vi "WVDIAL_1_AMCS_2.0_15m_res.vi"() -> ()   [LabVIEW 2012]
uses:
  <vilib>/Analysis/baseanly.llb/Mean (DBL).vi
  NCAR_DIAL_Labview/AMCS_Data.vi
  AmcsUsb.dll
  <vilib>/Analysis/NI_AALBase.lvlib
panel:
  out "x/y":dbl=nan
  out "Narrow Ratio":dbl(graph)=nan
  in  "Near Ch Offline mult":dbl=0.85
  out "size(s)":i32=5601
  in  "Channels":u32=4
  in  "Data Reads":i32=4
  out "Loop Count":i32=11
  in  "TC Start":i32=2 min=1 max=1894
  in  "TC Length":i32=15 min=2 max=280
  out "TC background sub over length":cluster{dbl, dbl, dbl, dbl}(graph)={0.0, 0.0, 1715.36170212766, 71287.61702127659}
  out "return type":i32
  out "Raw Uncorrected Return":u16[][](graph)
  in  "stop":bool
  out "Corrected Return":dbl[][](graph) caption="Corrected Signal"
  out "Max. Rep. Rate (Hz)":dbl=7091.695624423801
  out "Data Collection Time per Column":dbl=2.00004285
  out "Minimum Sync Pulse Period(µs)":dbl=141.01 format="%.2f"
  in  "y units":u16(ring) items=["Bin #", "Sampling Time(µs)", "Range(m)"]
  in  "Time Resolution Per Bin(ns)":u16=100 min=5 max=1063 step=1
  in  "Number of Accumulates":u32=14285 min=1 max=32767 step=1
  in  "Pulse A Polarity":enum16{"Low", "High"}(ring)=enum."High"
  in  "Sync Pulse Polarity":enum32{"Low", "High"}(ring)=enum."High"
  in  "Accumulation Delay(ns)":u16=10 min=10 max=1270 step=1
  in  "Pulse B Delay(ns)":u32=170000 min=80 max=327600 step=1
  in  "Pulse A Delay(ns)":u32=1040 min=80 max=327600
  in  "bins":u32=1400 min=2 max=4095 step=1
  out "y offset":u16=10
  in  "ns scale":u16=100
  in  "Pulse B Polarity":enum16{"Low", "High"}(ring)=enum."High"
  out "Running?":bool
  out "Device ID":u32
  out "Open?":bool=TRUE
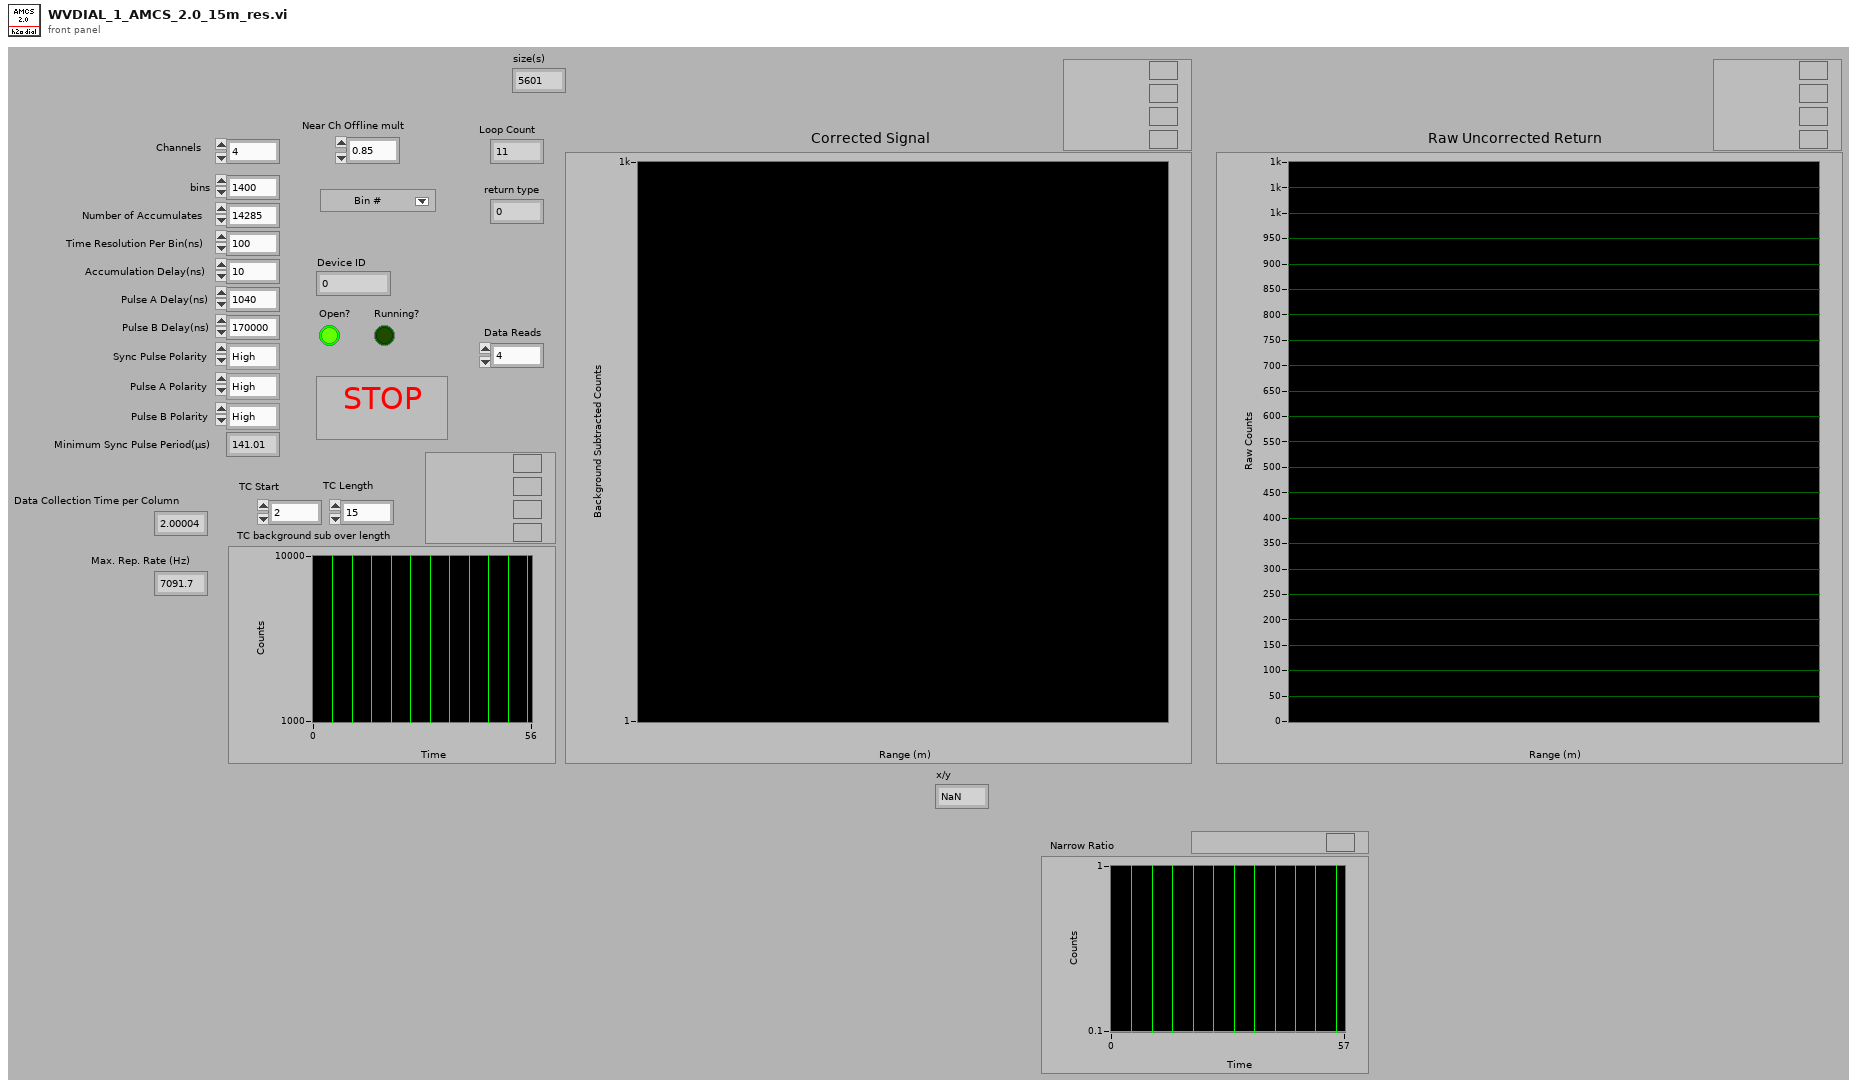
[diagram p1: front panel]
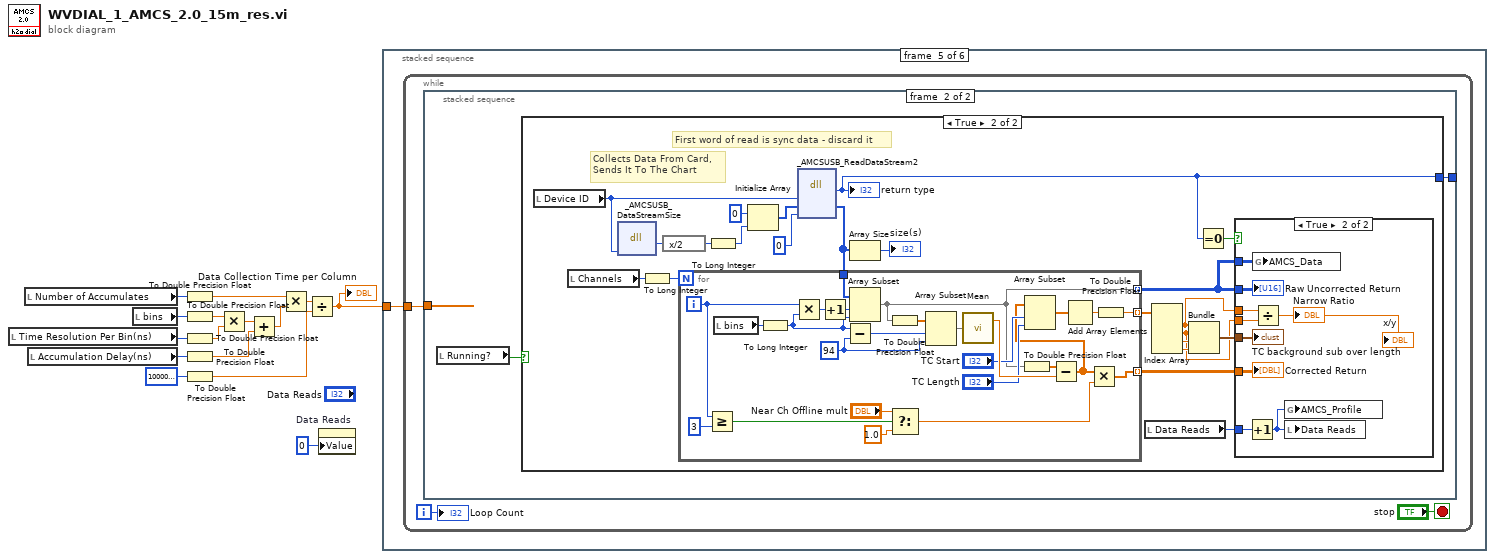
[diagram p0: block diagram]
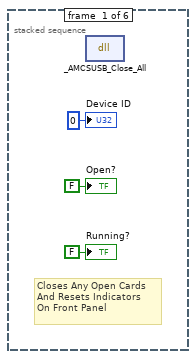
[diagram p2: hidden frame]
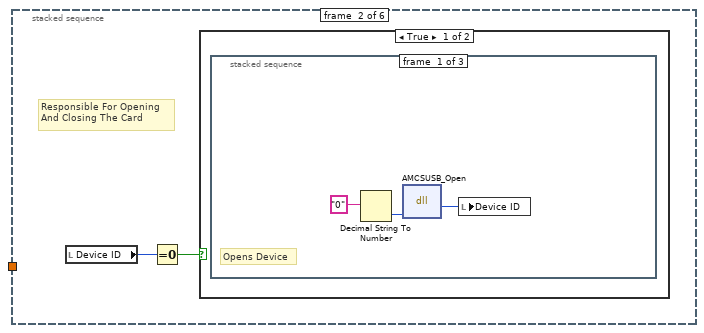
[diagram p3: hidden frame]
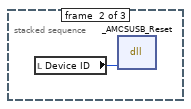
[diagram p4: hidden frame]
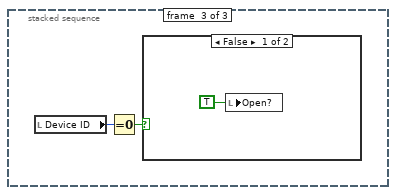
[diagram p5: hidden frame]
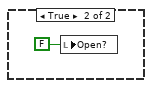
[diagram p6: hidden frame]
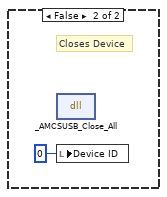
[diagram p7: hidden frame]
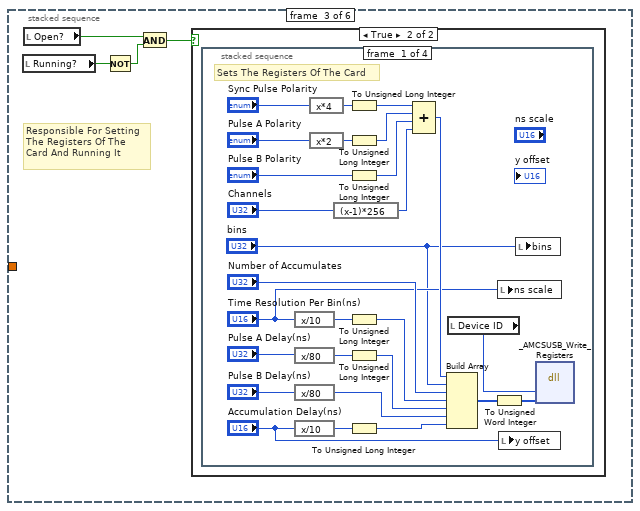
[diagram p8: hidden frame]
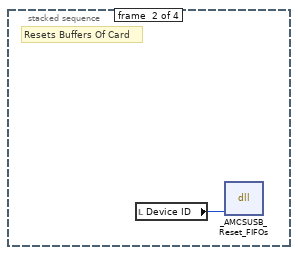
[diagram p10: hidden frame]
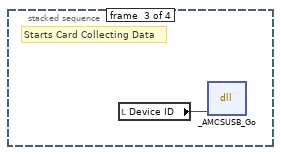
[diagram p11: hidden frame]
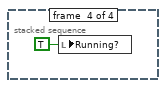
[diagram p12: hidden frame]
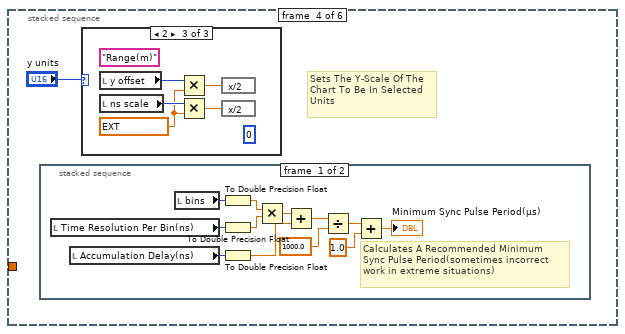
[diagram p13: hidden frame]
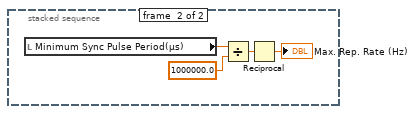
[diagram p14: hidden frame]
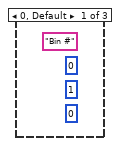
[diagram p15: hidden frame]
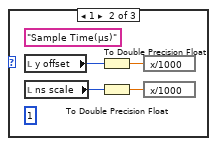
[diagram p16: hidden frame]
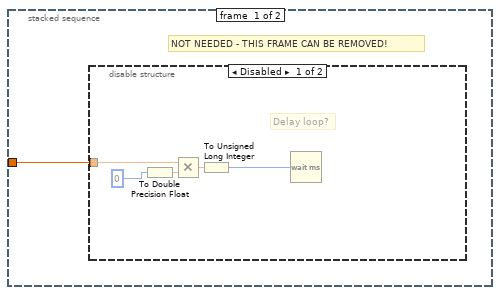
[diagram p17: hidden frame]
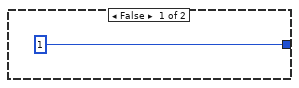
[diagram p19: hidden frame]
diagram:
  n1 = local read "Time Resolution Per Bin(ns)"() -> (w4:u16)
  n2 = local read "Number of Accumulates"() -> (w11:u32)
  n3 = local read "Accumulation Delay(ns)"() -> (w2:u16)
  n4 = local read "bins"() -> (w6:u32)
  n5 = To Double Precision Float(number=w11) -> (double precision float=w10:dbl)
  n6 = To Double Precision Float(number=w6) -> (double precision float=w5:dbl)
  n7 = To Double Precision Float(number=w4) -> (double precision float=w7:dbl)
  n8 = To Double Precision Float(number=w2) -> (double precision float=w3:dbl)
  n9 = To Double Precision Float(number=1000000000) -> (double precision float=w8:dbl)
  n10 = Multiply(x=w5, y=w7) -> (x*y=w15:dbl)
  n11 = Add(x=w15, y=w3) -> (x+y=w14:dbl)
  n12 = Multiply(x=w10, y=w14) -> (x*y=w13:dbl)
  n13 = Divide(x=w13, y=w8) -> (x/y=w12:dbl)
  "Data Collection Time per Column" <- w12
  n14 = property on="Data Reads" class="DigNum (strict)"("Value"=0 ("Data Reads")) -> ()  [unwired: 2 in, 2 out]
  n15 = stacked-sequence {
    tunnel: w12 -> [_ _ _ _ w90 _]
    frame #0 {
      # "Closes Any Open Cards\nAnd Resets Indicators\nOn Front Panel"
      n16 = dll-call lib="AmcsUsb.dll" fn="_AMCSUSB_Close_All" label="Close_All"() -> ()  [unwired: 4 in, 2 out]
      "Open?" <- FALSE ("Open?")
      "Device ID" <- u32 0 ("Device ID")
      "Running?" <- FALSE ("Running?")
    }
    frame #1 {
      # "Responsible For Opening\nAnd Closing The Card"
      n17 = local read "Device ID"() -> (w20:u32)
      n18 = Equal To 0?(x=w20) -> (x = 0?=w19:bool)
      n19 = case shown="True" w19 {
        frame True {
          # "Opens Device"
          n20 = stacked-sequence {
            frame #0 {
              n21 = Decimal String To Number(string="0" ("Device Number")) -> (number=w21:i32)  [unwired: 2 in, 1 out]
              n22 = dll-call lib="AmcsUsb.dll" fn="AMCSUSB_Open"("devnum"=w21) -> ("return type"=w22:u32)  [unwired: 4 in, 2 out]
              n23 = local write "Device ID"(w22) -> ()
            }
            frame #1 {
              n24 = local read "Device ID"() -> (w24:u32)
              n25 = dll-call lib="AmcsUsb.dll" fn="_AMCSUSB_Reset" label="Reset"("handle"=w24) -> ()  [unwired: 5 in, 2 out]
            }
            frame #2 {
              n26 = local read "Device ID"() -> (w25:u32)
              n27 = Equal To 0?(x=w25) -> (x = 0?=w26:bool)
              n28 = case shown="False" w26 {
                frame False {
                  n29 = local write "Open?"(TRUE ("Open?")) -> ()
                }
                frame True {
                  n30 = local write "Open?"(FALSE ("Open?")) -> ()
                }
              }
            }
          }
        }
        frame False {
          # "Closes Device"
          n31 = dll-call lib="AmcsUsb.dll" fn="_AMCSUSB_Close_All" label="Close_All"() -> ()  [unwired: 4 in, 2 out]
          n32 = local write "Device ID"(u32 0 ("Device ID")) -> ()
        }
      }
    }
    frame #2 {
      # "Responsible For Setting\nThe Registers Of The\nCard And Running It"
      n33 = local read "Running?"() -> (w32:bool)
      n34 = local read "Open?"() -> (w33:bool)
      n35 = Not(x=w32) -> (.not. x?=w31:bool)
      n36 = And(x=w33, y=w31) -> (x .and. y?=w30:bool)
      n37 = case shown="True" w30 {
        frame False {
        }
        frame True {
          n38 = stacked-sequence {
            frame #0 {
              # "Sets The Registers Of The Card"
              n39 = expression code="x/10"("Time Resolution Per Bin(ns)") -> (w38:u16)
              n40 = expression code="x/80"("Pulse A Delay(ns)") -> (w40:u32)
              n41 = expression code="x/80"("Pulse B Delay(ns)") -> (w60:u32)
              n42 = expression code="x/10"("Accumulation Delay(ns)") -> (w42:u16)
              n43 = expression code="x*4"("Sync Pulse Polarity") -> (w47:enum32{"Low", "High"})
              n44 = expression code="x*2"("Pulse A Polarity") -> (w46:enum16{"Low", "High"})
              n45 = expression code="(x-1)*256"("Channels") -> (w54:u32)
              n46 = To Unsigned Long Integer(number=w47) -> (unsigned 32bit integer=w48:u32)
              n47 = To Unsigned Long Integer(number=w46) -> (unsigned 32bit integer=w45:u32)
              n48 = To Unsigned Long Integer(number="Pulse B Polarity") -> (unsigned 32bit integer=w43:u32)
              n49 = To Unsigned Long Integer(number=w38) -> (unsigned 32bit integer=w37:u32)
              n50 = To Unsigned Long Integer(number=w40) -> (unsigned 32bit integer=w39:u32)
              n51 = To Unsigned Long Integer(number=w42) -> (unsigned 32bit integer=w41:u32)
              n52 = Compound Arithmetic op=ADD(w48, w45, w43, w54) -> (w59:u32)
              n53 = Build Array(w59, "bins", "Number of Accumulates", w37, w39, w60, w41) -> (w36:u32[])
              n54 = local read "Device ID"() -> (w52:u32)
              n55 = To Unsigned Word Integer(number=w36) -> (unsigned 16bit integer=w35:u16[])
              n56 = local write "ns scale"("Time Resolution Per Bin(ns)") -> ()
              n57 = local write "y offset"("Accumulation Delay(ns)") -> ()
              n58 = local write "bins"("bins") -> ()
              n59 = dll-call lib="AmcsUsb.dll" fn="_AMCSUSB_Write_Registers" label="Write_Registers"("handle"=w52, "registers"=w35) -> ()  [unwired: 6 in, 2 out]
            }
            frame #1 {
              # "Resets Buffers Of Card"
              n60 = local read "Device ID"() -> (w61:u32)
              n61 = dll-call lib="AmcsUsb.dll" fn="_AMCSUSB_Reset_FIFOs" label="Reset_FIFOs"("handle"=w61) -> ()  [unwired: 5 in, 2 out]
            }
            frame #2 {
              # "Starts Card Collecting Data"
              n62 = local read "Device ID"() -> (w62:u32)
              n63 = dll-call lib="AmcsUsb.dll" fn="_AMCSUSB_Go" label="Go"("handle"=w62) -> ()  [unwired: 5 in, 2 out]
            }
            frame #3 {
              n64 = local write "Running?"(TRUE) -> ()
            }
          }
        }
      }
    }
    frame #3 {
      # "Sets The Y-Scale Of The\nChart To Be In Selected\nUnits"
      n65 = stacked-sequence {
        frame #0 {
          # "Calculates A Recommended Minimum\nSync Pulse Period(sometimes incorrect\nwork in extreme situations)"
          n66 = local read "Time Resolution Per Bin(ns)"() -> (w71:u16)
          n67 = local read "Accumulation Delay(ns)"() -> (w73:u16)
          n68 = local read "bins"() -> (w72:u32)
          n69 = To Double Precision Float(number=w72) -> (double precision float=w74:dbl)
          n70 = To Double Precision Float(number=w71) -> (double precision float=w75:dbl)
          n71 = To Double Precision Float(number=w73) -> (double precision float=w76:dbl)
          n72 = Multiply(x=w74, y=w75) -> (x*y=w70:dbl)
          n73 = Add(x=w70, y=w76) -> (x+y=w68:dbl)
          n74 = Divide(x=w68, y=1000.0) -> (x/y=w67:dbl)
          n75 = Add(x=w67, y=1.0) -> (x+y=→"Minimum Sync Pulse Period(µs)":dbl)
        }
        frame #1 {
          n76 = local read "Minimum Sync Pulse Period(µs)"() -> (w78:dbl)
          n77 = Divide(x=w78, y=1000000.0) -> (x/y=w77:dbl)
          n78 = Reciprocal(x=w77) -> (1/x=→"Max. Rep. Rate (Hz)":dbl)
        }
      }
      n79 = case shown="2" "y units" {
        frame 0, Default {
          (unwired) u8 0 ("Y Scale.Format & Precision:Precision")
          (unwired) u16 1 ("Y Scale.Offset and Multiplier:Multiplier")
          (unwired) "Bin #" ("Y Scale.Name Label.Text")
          (unwired) u16 0 ("Y Scale.Offset and Multiplier:Offset")
        }
        frame 1 {
          (unwired) u8 1 ("Y Scale.Format & Precision:Precision")
          (unwired) "Sample Time(µs)" ("Y Scale.Name Label.Text")
          n80 = local read "y offset"() -> (w84:u16)
          n81 = local read "ns scale"() -> (w83:u16)
          n82 = To Double Precision Float(number=w84) -> (double precision float=w82:dbl)
          n83 = To Double Precision Float(number=w83) -> (double precision float=w81:dbl)
          n84 = expression code="x/1000"(w82) -> ()  [unwired: 1 out]
          n85 = expression code="x/1000"(w81) -> ()  [unwired: 1 out]
        }
        frame 2 {
          (unwired) u8 0 ("Y Scale.Format & Precision:Precision")
          w85 = ext 0.299792458 ("y")
          (unwired) "Range(m)" ("Y Scale.Name Label.Text")
          n86 = local read "y offset"() -> (w88:u16)
          n87 = local read "ns scale"() -> (w89:u16)
          n88 = Multiply(x=w88, y=w85) -> (x*y=w87:ext)
          n89 = Multiply(x=w89, y=w85) -> (x*y=w86:ext)
          n90 = expression code="x/2"(w87) -> ()  [unwired: 1 out]
          n91 = expression code="x/2"(w86) -> ()  [unwired: 1 out]
        }
      }
    }
    frame #4 {
      n92 = while {
        tunnel: w90 -> [w93]
        i -> [w91]
        stop <- "stop" stop-if-true
        n93 = stacked-sequence {
          tunnel: w93 -> [w94 _]
          tunnel: [_ w100] -> _
          frame #0 {
            # "NOT NEEDED - THIS FRAME CAN BE REMOVED!"
            n94 = disable-structure shown="Disabled" {
              disable-tunnel: w94 -> [w99 _]
              frame Disabled {
                # "Delay loop?"
                n95 = To Double Precision Float(number=0) -> (double precision float=w97:dbl)
                n96 = Multiply(x=w99, y=w97) -> (x*y=w96:dbl)
                n97 = To Unsigned Long Integer(number=w96) -> (unsigned 32bit integer=w95:u32)
                n98 = Wait (ms)(milliseconds to wait=w95) -> ()  [unwired: 1 out]
              }
              frame Enabled {
              }
            }
          }
          frame #1 {
            n99 = local read "Running?"() -> (w101:bool)
            n100 = case shown="True" w101 {
              tunnel: [1 ("return type") w109] -> w100
              frame False {
              }
              frame True {
                # "First word of read is sync data - discard it"
                # "Collects Data From Card,\nSends It To The Chart"
                n101 = local read "Device ID"() -> (w121:u32)
                n102 = local read "Channels"() -> (w113:u32)
                n103 = dll-call lib="AmcsUsb.dll" fn="_AMCSUSB_DataStreamSize" label="DataStreamSize"("handle"=w121) -> ("return type"=w120:u16)  [unwired: 4 in, 2 out]
                n104 = To Long Integer(number=w113) -> (32bit integer=w114:i32)
                n105 = expression code="x/2"(w120) -> (w119:u16)
                n106 = To Long Integer(number=w119) -> (32bit integer=w118:i32)
                n107 = Initialize Array(u32 0 ("element"), w118) -> (w122:u32[])
                n108 = dll-call lib="AmcsUsb.dll" fn="_AMCSUSB_ReadDataStream2" label="ReadDataStream2"("handle"=w121, "buffer"=w122, "BytesReturned"=u32 0) -> ("return type"=w109:i32, "buffer"=w108:u16[])  [unwired: 5 in, 2 out]
                "return type" <- w109
                n109 = for {
                  N: w114 -> [_]
                  tunnel: [w133] -> w112 mode=indexing
                  tunnel: [w132] -> w117 mode=indexing
                  tunnel: [w135] -> w106 mode=indexing
                  tunnel: w108 -> [w139]
                  i -> [w126]
                  w141 = 94 ("y")
                  n110 = Greater Or Equal?(x=w126, y=3) -> (x >= y?=w130:bool)
                  n111 = local read "bins"() -> (w145:u32)
                  n112 = To Long Integer(number=w145) -> (32bit integer=w143:i32)
                  n113 = Multiply(x=w126, y=w143) -> (x*y=w144:i32)
                  n114 = Increment(x=w144) -> (x+1=w138:i32)
                  n115 = Subtract(x=w143, y=w141) -> (x-y=w142:i32)
                  n116 = Array Subset(array=w139, index=w138, length=w143) -> (w135:u16[])
                  n117 = To Double Precision Float(number=w135) -> (double precision float=w134:dbl[])
                  n118 = Select(t="Near Ch Offline mult", s=w130, f=1.0 ("y")) -> (s? t:f=w127:dbl)
                  n119 = Array Subset(array=w134, index=w142, length=w141) -> (w149:dbl[])
                  n120 = call-poly <vilib>:"Mean.vi"("X"=w149) -> ("mean"=w147:dbl)  [unwired: 1 out]
                  n121 = To Double Precision Float(number=w135) -> (double precision float=w146:dbl[])
                  n122 = Subtract(x=w146, y=w147) -> (x-y=w125:dbl[])
                  n123 = Array Subset(array=w125, index="TC Start", length="TC Length") -> (w148:dbl[])
                  n124 = Add Array Elements(numeric array=w148) -> (sum=w140:dbl)
                  n125 = Multiply(x=w125, y=w127) -> (x*y=w132:dbl[])
                  n126 = To Double Precision Float(number=w140) -> (double precision float=w133:dbl)
                }
                n127 = Array Size(array=w108) -> (size(s)=→"size(s)":i32)
                n128 = local read "Data Reads"() -> (w105:i32)
                n129 = Index Array(array=w112) -> (element #1=w104:dbl, element #2=w103:dbl, element #3=w111:dbl, element #4=w110:dbl)  [unwired: 4 in]
                n130 = Bundle(w104, w103, w111, w110) -> (w115:cluster{dbl, dbl, dbl, dbl})  [unwired: 1 in]
                n131 = Equal To 0?(x=w109) -> (x = 0?=w116:bool)
                n132 = case shown="True" w116 {
                  tunnel: w117 -> [_ w158]
                  tunnel: w106 -> [_ w157]
                  tunnel: w115 -> [_ w156]
                  tunnel: w106 -> [_ w155]
                  tunnel: w105 -> [_ w154]
                  tunnel: w104 -> [_ w151]
                  tunnel: w103 -> [_ w150]
                  frame False {
                  }
                  frame True {
                    n133 = Increment(x=w154) -> (x+1=w153:i32)
                    n134 = global write "AMCS_Data.vi" "AMCS_Data"(w155) -> ()
                    n135 = Divide(x=w151, y=w150) -> (x/y=→"Narrow Ratio" →"x/y":dbl)
                    n136 = global write "AMCS_Data.vi" "AMCS_Profile"(w153) -> ()
                    n137 = local write "Data Reads"(w153) -> ()
                    "Corrected Return" <- w158
                    "Raw Uncorrected Return" <- w157
                    "TC background sub over length" <- w156
                  }
                }
              }
            }
          }
        }
        "Loop Count" <- w91
      }
    }
    frame #5 {
      # "Closes Any Open Cards\nAnd Resets Indicators\nOn Front Panel"
      n138 = dll-call lib="AmcsUsb.dll" fn="_AMCSUSB_Close_All" label="Close_All"() -> ()  [unwired: 4 in, 2 out]
      n139 = local write "Device ID"(u32 0 ("Device ID")) -> ()
      n140 = local write "Open?"(TRUE ("Open?")) -> ()
      n141 = local write "Running?"(FALSE ("Running?")) -> ()
    }
  }
